vi "Stop Core.vi"(10 "final error code":i32, 11 "Actor in":refnum<class "Actor1_GUI_G4_4.0.0.lvclass">) -> (3 "Actor out":refnum<class "Actor1_GUI_G4_4.0.0.lvclass">)   [LabVIEW 2020, in "Actor1_GUI_G4_4.0.0.lvlib" / "Actor1_GUI_G4_4.0.0.lvclass"]
doc: "(<B>Filename</B>: Actor Framework.lvlib:Actor.lvclass:Stop Core.vi)\n\nDefines what the actor does before it stops. Use the <B>final error code</B> input to determine whether the actor shut down in response to an error.\n\nBy default, this method does nothing. A descendant class may override it to define behavior, such as shutting down any processes the actor initiated in its override of the Actor Core method."
uses:
  Actor1_GUI_G4_4.0.0.lvclass
  <vilib>/ActorFramework/Actor/Actor.lvclass
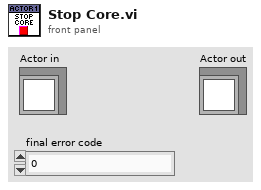
[diagram p1: front panel]
types:
  T1 = typedef "Actor1_GUI_G4_4.0.0.lvlib/Actor1_GUI_G4_4.0.0.lvclass/ObjectAttributes.ctl" = cluster{"LoopEvent":refnum<user-event>}
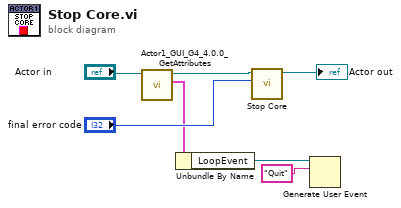
[diagram p0: block diagram]
diagram:
  n1 = call "Actor1_GUI_G4_4.0.0_GetAttributes.vi"("reference in"="Actor in") -> ("Data"=w2:T1, "reference out"=w4:refnum<class "Actor1_GUI_G4_4.0.0.lvclass">)  [unwired: 7 in, 2 out]
  n2 = Unbundle By Name(w2) -> ("LoopEvent"=w5:refnum<user-event>)
  n3 = call-parent "Stop Core.vi"("final error code"="final error code", "Actor in"=w4) -> ("Actor out"=→"Actor out":refnum<class "Actor1_GUI_G4_4.0.0.lvclass">)  [unwired: 9 in]
  n4 = Generate User Event(user event=w5, event data cluster="Quit" ("event data")) -> ()  [unwired: 2 in, 2 out]
